vi "teleportRobotsErForce.vi"(8 "error in (no error)":errorcluster, 9 "Original Array In":u8[](array[numeric]), 10 "robots":T1[](array[typedef]), 11 "Communication in":refnum<class "Communication.lvclass">) -> (0 "error out":errorcluster, 2 "teleportedRobotsArray":u8[](array[numeric]), 3 "Communication out":refnum<class "Communication.lvclass">)   [LabVIEW 2023, in "Communication.lvclass"]
uses:
  Communication.lvclass
  grSim Packet Command UDP Test Folder/grSim/grSim RobotReplacement.ctl
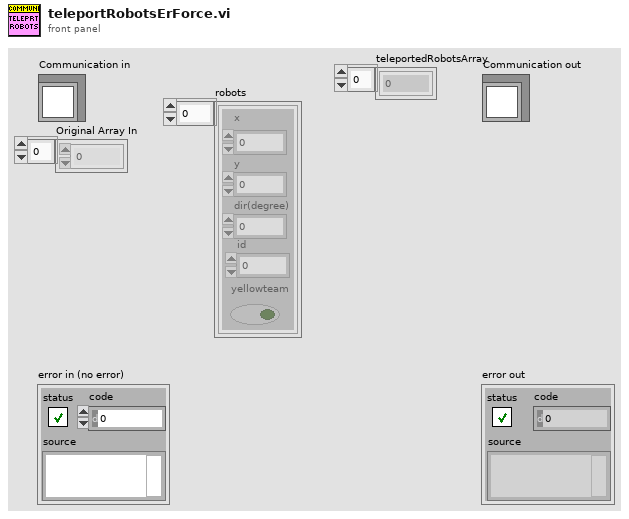
[diagram p1: front panel]
types:
  T1 = typedef "grSim RobotReplacement.ctl" = cluster{"x":dbl, "y":dbl, "dir(degree)":dbl, "yellowteam":bool, "id":u32}
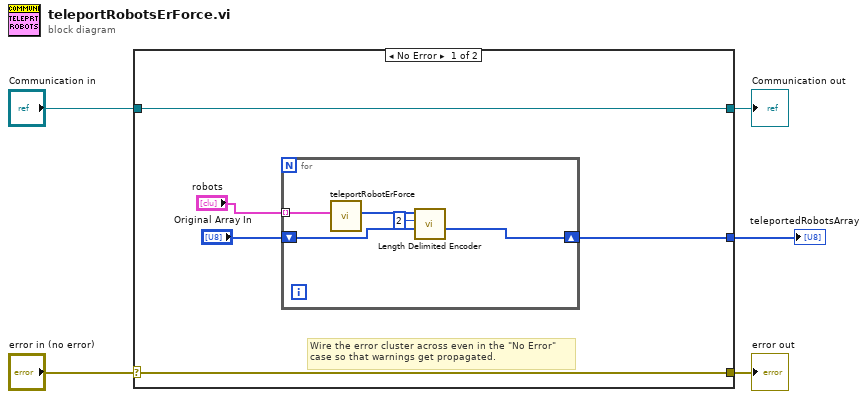
[diagram p0: block diagram]
diagram:
  n1 = case shown="No Error" "error in (no error)" {
    selector: "error in (no error)" -> [w9 w17]
    tunnel: [w9 w17] -> w4
    tunnel: [w10 w16] -> w2
    tunnel: "Communication in" -> [w10 w16]
    tunnel: [w6 _] -> w1
    frame No Error {
      # "Wire the error cluster across even in the \"No Error\"\ncase so that warnings get propagated."
      n2 = for {
        shift-right: [w14] -> w6
        shift-left: "Original Array In" -> [w13]
        tunnel: "robots" -> [w12] mode=indexing
        n3 = call "teleportRobotErForce.vi"("robot"=w12) -> ("TeleportRobotArray"=w15:u8[])  [unwired: 8 in, 2 out]
        n4 = call "Length Delimited Encoder.vi"("Original Array In"=w13, "Key"=u32 2, "Array In to be added"=w15) -> ("Array"=w14:u8[])  [unwired: 8 in]
      }
    }
    frame Error {
    }
  }
  "error out" <- w4
  "Communication out" <- w2
  "teleportedRobotsArray" <- w1
